vi "LineScanStatus.vi"(1 "Get/Set":bool, 2 "Linescan Status (input)":T1 {"new plane step"."z" format="%.2f"; "new plane step"."y" format="%.2f"; "new plane step"."x" format="%.2f"; "new line step"."z" format="%.2f"; "new line step"."y" format="%.2f"; "new line step"."x" format="%.2f"}) -> (0 "Linescan Status (output)":T1 {"new plane step"."z" format="%.2f"; "new plane step"."y" format="%.2f"; "new plane step"."x" format="%.2f"; "new line step"."z" format="%.2f"; "new line step"."y" format="%.2f"; "new line step"."x" format="%.2f"})   [LabVIEW 2009]
uses:
  LineScanStatus.ctt
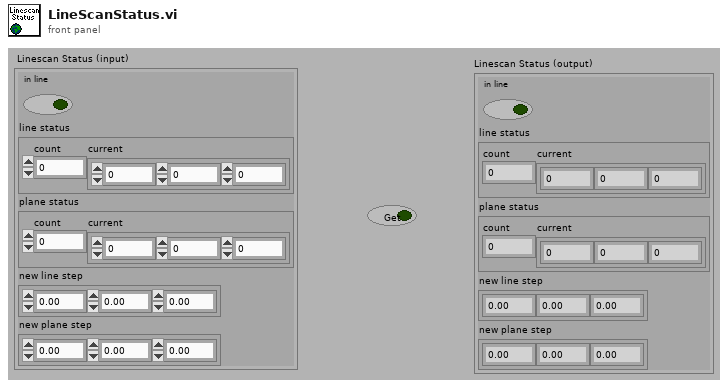
[diagram p1: front panel]
types:
  T1 = typedef "LineScanStatus.ctt" = cluster{"in line":bool, "line status":cluster{"count":u32, "current":cluster{"x":u32, "y":u32, "z":u32}}, "plane status":cluster{"count":u32, "current":cluster{"x":u32, "y":u32, "z":u32}}, "new line step":cluster{"x":dbl, "y":dbl, "z":dbl}, "new plane step":cluster{"x":dbl, "y":dbl, "z":dbl}}
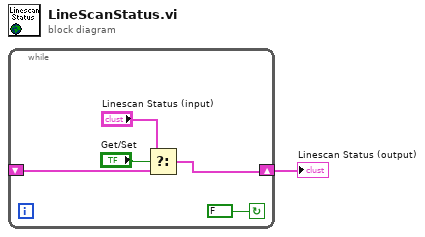
[diagram p0: block diagram]
diagram:
  n1 = while {
    shift-right: [w4] -> w1
    shift-left: _ -> [w5]
    stop <- FALSE continue-if-true
    n2 = Select(t="Linescan Status (input)", s="Get/Set", f=w5) -> (s? t:f=w4:T1)
  }
  "Linescan Status (output)" <- w1
